vi "Process Job.vi"(8 "error in (no error)":errorcluster, 10 "Job":refnum<class>, 11 "Worker In":refnum<class "Worker.lvclass">) -> (0 "error out":errorcluster, 3 "Worker Out":refnum<class "Worker.lvclass">)   [LabVIEW 2020, in "Worker.lvclass"]
uses:
  Worker.lvclass
  C:/Program Files (x86)/National Instruments/LabVIEW 2020/vi.lib/Astemes/Triarc Framework/Process/Process.lvclass
  <vilib>/Astemes/Triarc Framework/Process/Process.lvclass/Process.ctl
  <vilib>/Astemes/Triarc Framework/Process/Private/SubVIs/Handle Debug Data.vi
  <vilib>/Astemes/Triarc Framework/Logging/Log Debug.vi
  <vilib>/AdvancedString/1D String Array to Delimited String.vi
  <vilib>/Utility/High Resolution Relative Seconds.vi
  <vilib>/Astemes/Triarc Framework/Process/Public/Read Name.vi
  <vilib>/Astemes/Triarc Framework/Callback/Callback.lvclass
  <vilib>/Astemes/Triarc Framework/Process/Process.lvclass
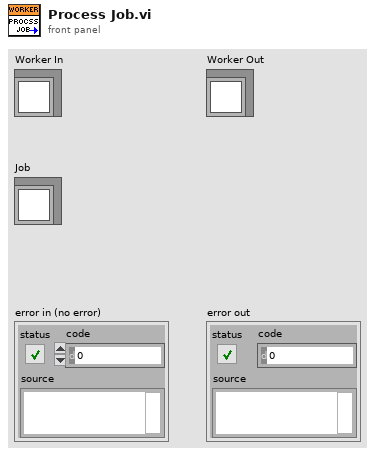
[diagram p1: front panel]
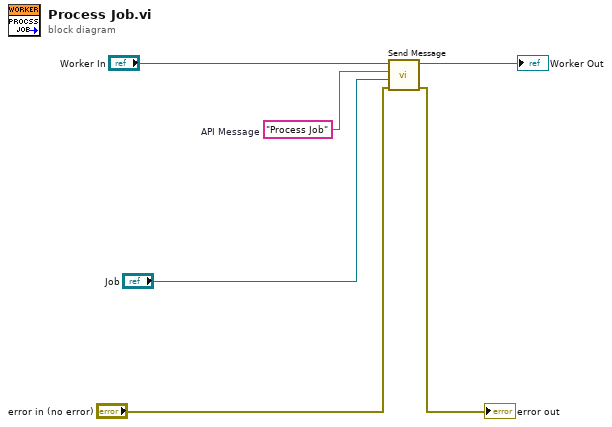
[diagram p0: block diagram]
diagram:
  w3 = "Process Job"  # API Message
  n1 = call <vilib>:"Send Message.vi"("error in (no error)"="error in (no error)", "Message Data"="Job", "Message"=w3, "Process In"="Worker In") -> ("error out"=→"error out":errorcluster, "Process Out"=→"Worker Out":refnum<class "Worker.lvclass">)  [unwired: 6 in]
